vi "Do.vi"(8 "error in (no error)":errorcluster, 10 "Actor in":refnum<class "Actor.lvclass">, 11 "Configure Standard Waveform [STD] Msg":refnum<class "Configure Standard Waveform [STD] Msg.lvclass">) -> (0 "error out":errorcluster, 2 "Actor out":refnum<class "Actor.lvclass">)   [LabVIEW 2015, in "CS++Fgen.lvlib" / "Configure Standard Waveform [STD] Msg.lvclass"]
doc: "This VI delivers the message to the actor by calling the appropriate method(s) on the actor."
uses:
  Configure Standard Waveform [STD] Msg.lvclass
  <vilib>/ActorFramework/Actor/Actor.lvclass
  CS++Fgen/CS++Fgen.lvclass
  CSPP_Core/Actors/CS++PVMonitor Messages/CS++PVUpdate Msg/CS++PVUpdate Msg.lvclass/CS++PVUpdate Msg.ctl
  CSPP_Core/Classes/CS++ProcessVariables/ProcessVariable/PV.lvclass/PV.ctl
  Configure Standard Waveform [STD] Msg.lvclass/Configure Standard Waveform [STD] Msg.ctl
  CSPP_Core/Classes/CS++ProcessVariables/ProcessVariable/PV.lvclass
  CSPP_Core/Actors/CS++PVMonitor Messages/CS++PVUpdate Msg/CS++PVUpdate Msg.lvclass
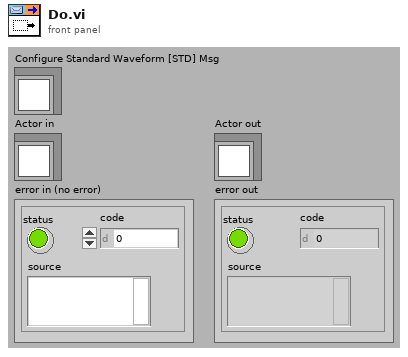
[diagram p1: front panel]
types:
  T1 = cluster{"channel name (\"CHANNEL1\")":string, "waveform (Sine)":i32, "frequency (1000.0 Hz)":dbl[unit], "start phase (0.00 Degrees)":dbl[unit], "amplitude (1.00 V)":dbl[unit], "dc offset (0.00 V)":dbl[unit]}
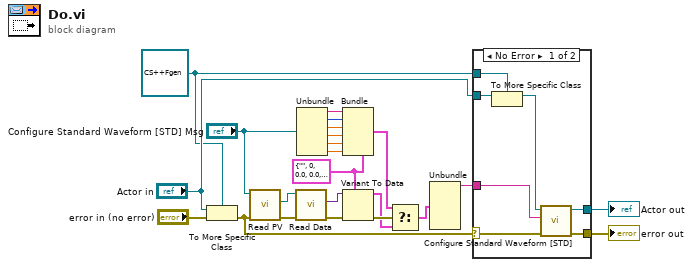
[diagram p0: block diagram]
diagram:
  w15 = T1 {"channel name (\"CHANNEL1\")"="", "waveform (Sine)"=0, "frequency (1000.0 Hz)"=0.0, "start phase (0.00 Degrees)"=0.0, "amplitude (1.00 V)"=0.0, "dc offset (0.00 V)"=0.0} ("Type")
  w19 = refnum<class "CS++Fgen.lvclass"> refnum ("Actor in")
  n1 = To More Specific Class(target class=w19, reference="Actor in", error in="error in (no error)") -> (error out=w8:errorcluster)  [unwired: 1 out]
  n2 = call "Read PV.vi"("error in (no error)"=w8, "CS++PVUpdate Msg in"="Configure Standard Waveform [STD] Msg") -> ("error out"=w18:errorcluster, "PV"=w14:refnum<class "PV.lvclass">)  [unwired: 7 in, 1 out]
  n3 = call "Read Data.vi"("error in (no error)"=w18, "PV in"=w14) -> ("error out"=w12:errorcluster, "Data"=w13:variant)  [unwired: 7 in, 1 out]
  n4 = Unbundle ("Pre-Unbundler")("Configure Standard Waveform [STD] Msg") -> (w6:string, w5:i32, w4:dbl[unit], w3:dbl[unit], w2:dbl[unit], w1:dbl[unit])
  n5 = Bundle ("Pre-Bundler")(cluster=w15, "channel name (\"CHANNEL1\")"=w6, "waveform (Sine)"=w5, "frequency (1000.0 Hz)"=w4, "start phase (0.00 Degrees)"=w3, "amplitude (1.00 V)"=w2, "dc offset (0.00 V)"=w1) -> (w16:T1)
  n6 = Variant To Data(error in=w12, type=w15, Variant=w13) -> (data=w10:T1, error out=w17:errorcluster)
  n7 = Select ("MainSelect")(t=w16, s=w17, f=w10) -> (s? t:f=w11:T1)
  n8 = Unbundle ("Main-Unbundler")(w11) -> ("channel name (\"CHANNEL1\")"=w7:string)  [unwired: 5 out]
  n9 = case shown="No Error" w8 {
    selector: w8 -> [w28 w32]
    tunnel: [w30 w32] -> w22
    tunnel: [w29 w31] -> w21
    tunnel: "Actor in" -> [w27 w31]
    tunnel: w19 -> [w26 _]
    tunnel: w7 -> [w24 _]
    frame No Error {
      n10 = To More Specific Class(target class=w26, reference=w27) -> (specific class reference=w25:refnum<class "CS++Fgen.lvclass">)  [unwired: 1 in, 1 out]
      n11 = call "Configure Standard Waveform [STD].vi"("error in (no error)"=w28, "channel name (\"CHANNEL1\")"=w24, "CS++Fgen in"=w25) -> ("error out"=w30:errorcluster, "CS++Fgen out"=w29:refnum<class "CS++Fgen.lvclass">)  [unwired: 7 in]
    }
    frame Error {
    }
  }
  "error out" <- w22
  "Actor out" <- w21
